vi "DrawString.vi"(4 "SpaceTilecode(206)":u32=206, 6 "ColorToReplace (7=white)":fxp<+,3,3>=7.0, 7 "Color (7=white)":fxp<+,3,3>=7.0, 8 "error in (no error)":errorcluster, 9 "Coordinate":T1, 10 "String":string, 11 "RT_Game.lvlib:Game.lvclass":refnum<class "Game.lvclass">) -> (0 "error out":errorcluster, 3 "RT_Game.lvlib:Game.lvclass 2":refnum<class "Game.lvclass">)   [LabVIEW 2019, in "RT_Game.lvlib" / "Game.lvclass"]
uses:
  Game.lvclass
  Coordinate.ctl
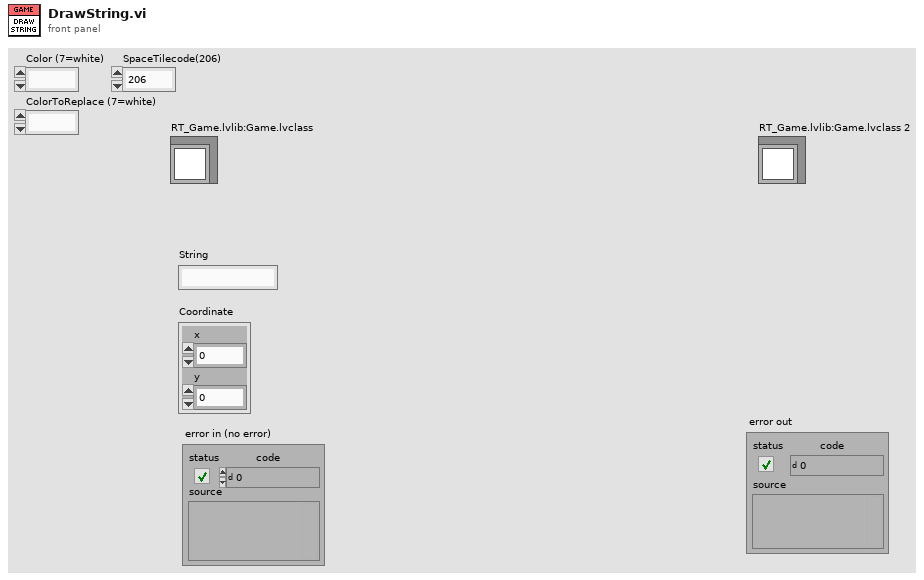
[diagram p1: front panel]
types:
  T1 = typedef "RT_Game.lvlib/Game.lvclass/Coordinate.ctl" = cluster{"x":dbl, "y":dbl}
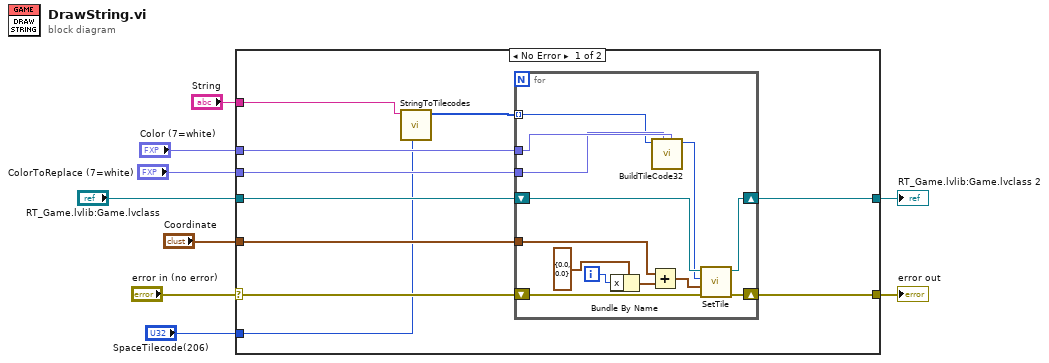
[diagram p0: block diagram]
diagram:
  n1 = case shown="No Error" "error in (no error)" {
    selector: "error in (no error)" -> [w19 w34]
    tunnel: [w18 w34] -> w8
    tunnel: [w16 w33] -> w6
    tunnel: "RT_Game.lvlib:Game.lvclass" -> [w17 w33]
    tunnel: "Coordinate" -> [w15 _]
    tunnel: "String" -> [w11 _]
    tunnel: "Color (7=white)" -> [w14 _]
    tunnel: "ColorToReplace (7=white)" -> [w13 _]
    tunnel: "SpaceTilecode(206)" -> [w10 _]
    frame No Error {
      n2 = call "StringToTilecodes.vi"("SpaceTilecode(206)"=w10, "String"=w11) -> ("Tilecodes"=w12:u32[])  [unwired: 9 in]
      n3 = for {
        shift-right: [w31] -> w18
        shift-left: w19 -> [w32]
        shift-right: [w29] -> w16
        shift-left: w17 -> [w30]
        tunnel: w15 -> [w28]
        tunnel: w14 -> [w23]
        tunnel: w13 -> [w22]
        tunnel: w12 -> [w21] mode=indexing
        i -> [w24]
        n4 = Bundle By Name(cluster=T1 {"x"=0.0, "y"=0.0} ("y"), "x"=w24) -> (w25:T1)
        n5 = Add(x=w28, y=w25) -> (x+y=w27:T1)
        n6 = call "BuildTileCode32.vi"("replacecolor"=w23, "color_to_replace"=w22, "Tilenumber"=w21) -> ("TileCode"=w20:u32)  [unwired: 8 in]
        n7 = call "SetTile.vi"("error in (no error)"=w32, "Coordinates"=w27, "TileNumber"=w20, "Game in"=w30) -> ("error out"=w31:errorcluster, "Game out"=w29:refnum<class "Game.lvclass">)  [unwired: 6 in]
      }
    }
    frame Error {
    }
  }
  "RT_Game.lvlib:Game.lvclass 2" <- w6
  "error out" <- w8
